vi "SeCrTs-String combo refX.vi"(8 "error out":errorcluster, 11 "Ctrl ref":refnum<vi>[](array[refnum])) -> (0 "error out 2":errorcluster)   [LabVIEW 2022 SP3]
panel:
  in  "Signal names":string[][](array[string])
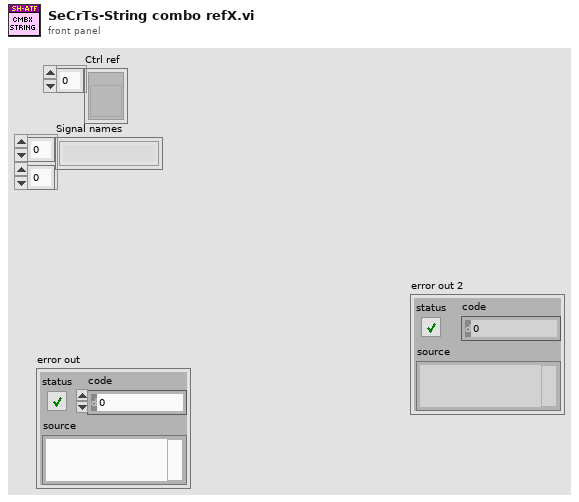
[diagram p1: front panel]
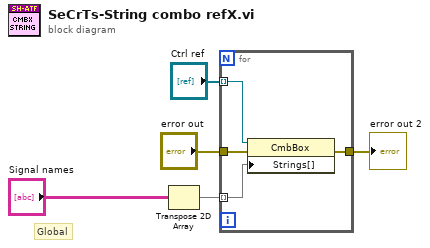
[diagram p0: block diagram]
diagram:
  # "Global"
  n1 = Transpose 2D Array(2D array="Signal names") -> (transposed array=w2:string[][])
  n2 = for {
    tunnel: "Ctrl ref" -> [w9] mode=indexing
    tunnel: w2 -> [w6] mode=indexing
    tunnel: [w8] -> w3
    tunnel: "error out" -> [w7]
    n3 = property class="CmbBox"(reference=w9, error in=w7, "Strings[]"=w6) -> (error out=w8:errorcluster)  [unwired: 1 out]
  }
  "error out 2" <- w3
